vi "Get Dual Exposure Times.vi"(8 "error in (no error)":errorcluster, 10 "exposure2":sgl, 11 "exposure1":sgl) -> (0 "error out":errorcluster, 1 "function return":u32, 2 "exposure2 out":sgl, 3 "exposure1 out":sgl)   [LabVIEW 2014, in "atmcd32d.lvlib"]
doc: "unsigned int WINAPI GetDualExposureTimes(float * exposure1, float * exposure2);"
uses:
  atmcd32d.lvlib
  atmcd32d.dll
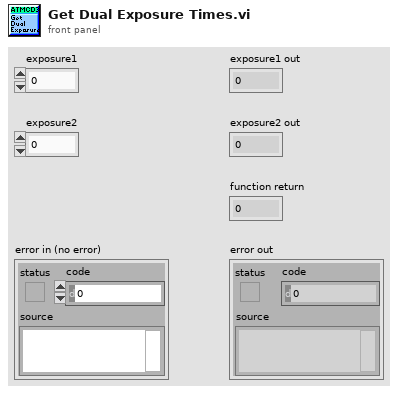
[diagram p1: front panel]
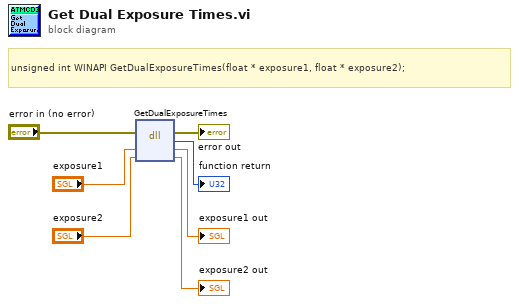
[diagram p0: block diagram]
diagram:
  # "unsigned int WINAPI GetDualExposureTimes(float * exposure1, float * exposure2);"
  n1 = dll-call lib="C:/Users/Bakir/Documents/Lambda2-Testing/lib/Andorlib/atmcd32d.*" fn="GetDualExposureTimes"(error in="error in (no error)", "exposure1"="exposure1", "exposure2"="exposure2") -> (error out=→"error out":errorcluster, →"function return":u32, "exposure1"=→"exposure1 out":sgl, "exposure2"=→"exposure2 out":sgl)  [unwired: 2 in, 1 out]
